vi "Servo MSMT SpecAn Create Evaluations.vi"(8 "error in (no error)":errorcluster, 11 "Servo MSMT in":refnum<class "Servo MSMT.lvclass">) -> (0 "error out":errorcluster, 2 "Specan Evaluations":T1[](array[typedef]) {"Low Limit" format="%#_13g"; "SI Scaling" items=["femto"=-15, "pico"=-12, "nano"=-9, "micro"=-6, "milli"=-3, "percent"=-2, ""=0, "kilo"=3, "mega"=6, "giga"=9, "tera"=12]}, 3 "Servo MSMT out":refnum<class "Servo MSMT.lvclass">)   [LabVIEW 2018, in "Servo MSMT.lvlib" / "Servo MSMT.lvclass"]
uses:
  Servo MSMT.lvclass
  C:/Sequence Automation/Plugins/Measurement Interface.lvlibp/Measurement Interface.lvclass
  Plugins/TestStand API Tools (TSAT).lvlibp/Evaluation Actions/Includes/Controls/TSAT Evaluation.ctl
  Plugins/TestStand API Tools (TSAT).lvlibp/Evaluation Actions/Includes/Controls/TSAT Eval SI Unit Scaling.ctl
  Plugins/TestStand API Tools (TSAT).lvlibp/Evaluation Actions/Includes/Controls/TSAT Evaluation Type.ctl
  Plugins/SeqAuto IEvaluation.lvlibp/SeqAuto IEvaluation.lvclass
  Servo MSMT.lvclass/Servo MSMT.ctl
  Protected Methods/Read DC Pins.vi
  Protected Methods/Read Servo Measurements.vi
  Plugins/SeqAuto Evaluations.lvlibp/LTE Evaluations/LTE_ACP/LTE_ACP.lvclass
  C:/Sequence Automation/Plugins/SeqAuto IEvaluation.lvlibp/SeqAuto IEvaluation.lvclass
  Plugins/SeqAuto Evaluations.lvlibp/LTE Evaluations/LTE_OBW/LTE_OBW.lvclass
  Plugins/SeqAuto Evaluations.lvlibp/SpecAn Evaluations/SpecAn CHP/SpecAn_CHP.lvclass
  Evaluations/SpecAn Evaluations/SpecAn AMPM/SpecAn_AMPM.lvclass
  Plugins/SeqAuto Evaluations.lvlibp/LTE Evaluations/LTE_SEM/LTE_SEM.lvclass
  Plugins/SeqAuto Evaluations.lvlibp/Servo/Servo Gain/Servo Gain.lvclass
  Plugins/SeqAuto Evaluations.lvlibp/PA Evaluations/PAE/PAE.lvclass
  Plugins/SeqAuto Evaluations.lvlibp/LTE Evaluations/LTE_ModAcc/LTE_ModAcc.lvclass
  Plugins/SeqAuto Evaluations.lvlibp/SpecAn Evaluations/SpecAn IM3/SpecAn_IM3.lvclass
  Plugins/SeqAuto Evaluations.lvlibp/DC Evaluations/DC_IDD.lvclass
  Plugins/Measurement Interface.lvlibp/Private Methods/Measurement Name/Read Measurement Name.vi
  Plugins/Measurement Interface.lvlibp/Private Methods/Measurement Parameters/Read Measurement Parameters.vi
  Plugins/String Database.lvlibp/String Database.lvclass
  Plugins/Test Number and Bin Generator.lvlibp/Test Number and Bin Generator/Test Number and Bin Generator.lvclass
  Plugins/TestStand API Tools (TSAT).lvlibp/Evaluation Actions/TSAT Evaluation Actions.lvlib
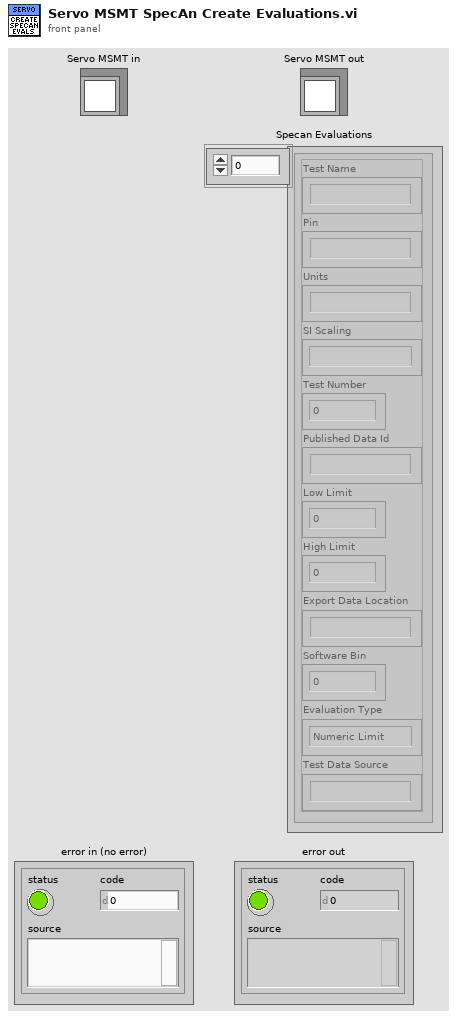
[diagram p1: front panel]
types:
  T1 = typedef "TestStand API Tools (TSAT).lvlibp/TSAT Evaluation Actions.lvlib/TSAT Evaluation.ctl" = cluster{"Test Name":string, "Pin":string, "Units":string, "SI Scaling":T2, "Test Number":i32, "Published Data Id":string, "Low Limit":dbl, "High Limit":dbl, "Export Data Location":string, "Software Bin":i64, "Evaluation Type":T3, "Test Data Source":string}
  T2 = typedef "TestStand API Tools (TSAT).lvlibp/TSAT Evaluation Actions.lvlib/TSAT Eval SI Unit Scaling.ctl" = i16
  T3 = typedef "TestStand API Tools (TSAT).lvlibp/TSAT Evaluation Actions.lvlib/TSAT Evaluation Type.ctl" = enum16{"Numeric Limit", "Pass/Fail", "None"}
  T4 = typedef "Test Number and Bin Generator.lvlibp/Test Number and Bin Generator.lvclass/Session Handle.ctl" = refnum<data-value>
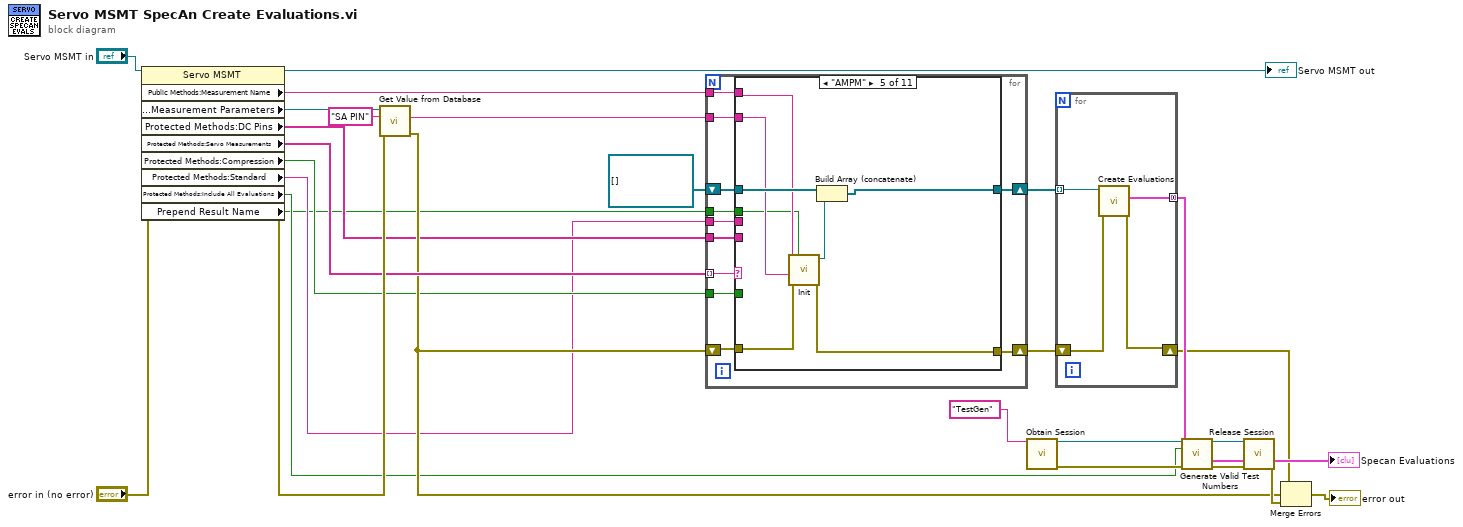
[diagram p0: block diagram]
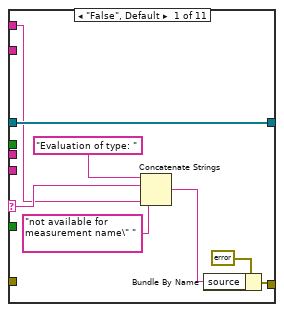
[diagram p2: hidden frame]
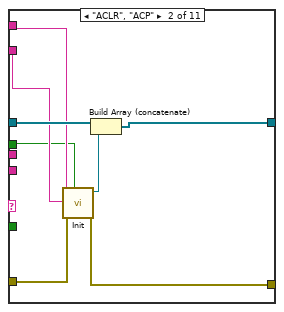
[diagram p3: hidden frame]
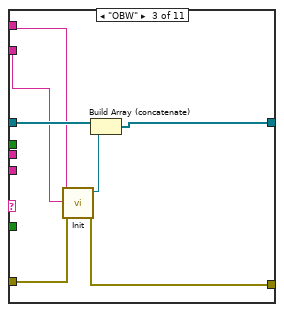
[diagram p4: hidden frame]
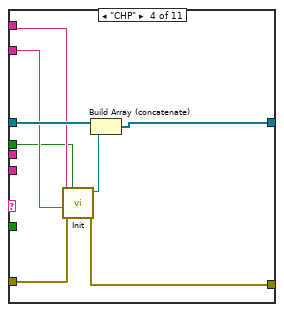
[diagram p5: hidden frame]
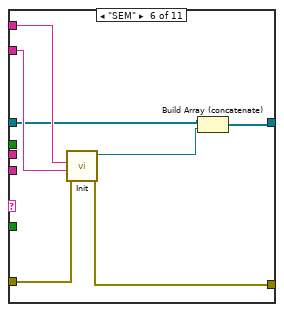
[diagram p6: hidden frame]
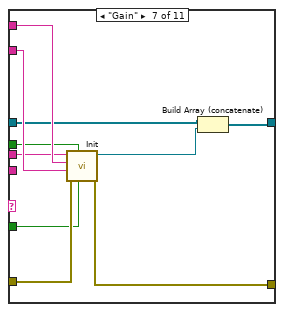
[diagram p7: hidden frame]
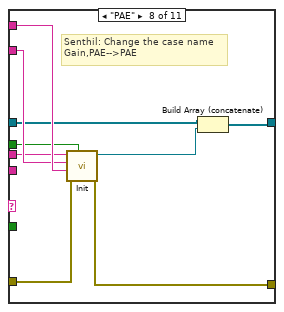
[diagram p8: hidden frame]
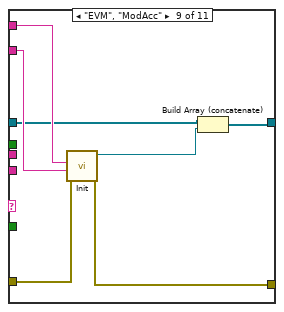
[diagram p9: hidden frame]
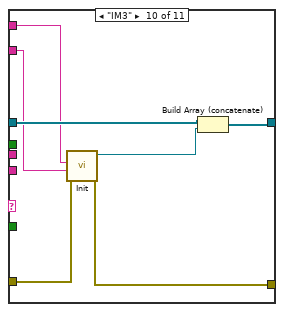
[diagram p10: hidden frame]
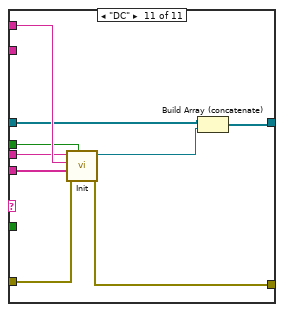
[diagram p11: hidden frame]
diagram:
  n1 = property class="Servo MSMT"(reference="Servo MSMT in", error in="error in (no error)") -> (reference out=→"Servo MSMT out":refnum<class "Servo MSMT.lvclass">, error out=w12:errorcluster, "Public Methods:Measurement Name"=w14:string, "Protected Methods:Measurement Parameters"=w18:refnum<class "String Database.lvclass">, "Protected Methods:DC Pins"=w5:string[], "Protected Methods:Servo Measurements"=w9:string[], "Protected Methods:Compression"=w4:bool, "Protected Methods:Standard"=w3:string, "Protected Methods:Include All Evaluations"=w2:bool, "Prepend Result Name"=w1:bool)
  n2 = call "Get Value from Database.vi"("error in (no error)"=w12, "Entry Name"="SA PIN", "Message in"=w18) -> ("error out"=w8:errorcluster, "Entry Value"=w17:string)  [unwired: 5 in, 2 out]
  n3 = for {
    tunnel: w17 -> [w39]
    tunnel: w14 -> [w38]
    shift-right: [w36] -> w16
    shift-left: refnum<class "SeqAuto IEvaluation.lvclass">[] [] -> [w37]
    tunnel: w9 -> [w35] mode=indexing
    shift-right: [w33] -> w7
    shift-left: w8 -> [w34]
    tunnel: w5 -> [w32]
    tunnel: w3 -> [w31]
    tunnel: w4 -> [w30]
    tunnel: w1 -> [w29]
    n4 = case shown="\"AMPM\"" w35 {
      selector: w35 -> [w43 _ _ _ _ _ _ _ _ _ _]
      tunnel: w39 -> [_ w49 w56 w64 w72 w84 w94 w103 w110 w112 _]
      tunnel: w38 -> [w41 w50 w57 w65 w73 w85 w95 w104 w111 w113 w127]
      tunnel: [w47 w55 w62 w70 w78 w79 w89 w98 w105 w114 w122] -> w36
      tunnel: w37 -> [w47 w54 w61 w69 w77 w81 w91 w100 w107 w116 w124]
      tunnel: w34 -> [_ w52 w59 w67 w75 w83 w93 w102 w109 w118 w126]
      tunnel: [w45 w51 w58 w66 w74 w82 w92 w101 w108 w117 w125] -> w33
      tunnel: w32 -> [_ _ _ _ _ _ _ _ _ _ w121]
      tunnel: w31 -> [_ _ _ _ _ _ w88 w97 _ _ w120]
      tunnel: w30 -> [_ _ _ _ _ _ w87 _ _ _ _]
      tunnel: w29 -> [_ w48 _ w63 w71 _ w86 w96 _ _ w119]
      frame "False", Default {
        n5 = Concatenate Strings("Evaluation of type: " ("source"), w43, "not available for measurement name\" " ("source"), w41) -> (w40:string)
        n6 = Bundle By Name(cluster=errorcluster {"status"=TRUE, "code"=7777, "source"=""} ("error out"), "source"=w40) -> (w45:errorcluster)
      }
      frame "ACLR", "ACP" {
        n7 = call "Init.vi"("Prepend Result Name"=w48, "error in (no error)"=w52, "SA Pin"=w49, "Measurement Name"=w50) -> ("error out"=w51:errorcluster, "LTE_ACP out"=w53:refnum<class "LTE_ACP.lvclass">)  [unwired: 6 in]
        n8 = Build Array (concatenate)(w54, w53) -> (w55:refnum<class "SeqAuto IEvaluation.lvclass">[])
      }
      frame "OBW" {
        n9 = call "Init.vi"("error in (no error)"=w59, "SA Pin"=w56, "Measurement Name"=w57) -> ("error out"=w58:errorcluster, "LTE_OBW out"=w60:refnum<class "LTE_OBW.lvclass">)  [unwired: 7 in]
        n10 = Build Array (concatenate)(w61, w60) -> (w62:refnum<class "SeqAuto IEvaluation.lvclass">[])
      }
      frame "CHP" {
        n11 = call "Init.vi"("Prepend Result Name"=w63, "error in (no error)"=w67, "SA Pin"=w64, "Measurement Name"=w65) -> ("error out"=w66:errorcluster, "SpecAn_CHP out"=w68:refnum<class "SpecAn_CHP.lvclass">)  [unwired: 6 in]
        n12 = Build Array (concatenate)(w69, w68) -> (w70:refnum<class "SeqAuto IEvaluation.lvclass">[])
      }
      frame "AMPM" {
        n13 = call "Init.vi"("Prepend Result Name"=w71, "error in (no error)"=w75, "SA Pin"=w72, "Measurement Name"=w73) -> ("error out"=w74:errorcluster, "SpecAn_AMPM out"=w76:refnum<class "SpecAn_AMPM.lvclass">)  [unwired: 6 in]
        n14 = Build Array (concatenate)(w77, w76) -> (w78:refnum<class "SeqAuto IEvaluation.lvclass">[])
      }
      frame "SEM" {
        n15 = call "Init.vi"("error in (no error)"=w83, "SA Pin"=w84, "Measurement Name"=w85) -> ("error out"=w82:errorcluster, "LTE_SEM out"=w80:refnum<class "LTE_SEM.lvclass">)  [unwired: 7 in]
        n16 = Build Array (concatenate)(w81, w80) -> (w79:refnum<class "SeqAuto IEvaluation.lvclass">[])
      }
      frame "Gain" {
        n17 = call "Init.vi"("Compression?"=w87, "Prepend Result Name"=w86, "error in (no error)"=w93, "SA Pin"=w94, "Measurement Name"=w95, "Standard"=w88) -> ("error out"=w92:errorcluster, "Servo Gain out"=w90:refnum<class "Servo Gain.lvclass">)  [unwired: 4 in]
        n18 = Build Array (concatenate)(w91, w90) -> (w89:refnum<class "SeqAuto IEvaluation.lvclass">[])
      }
      frame "PAE" {
        # "Senthil: Change the case name\nGain,PAE-->PAE"
        n19 = call "Init.vi"("Prepend Result Name"=w96, "error in (no error)"=w102, "Measurement Name"=w104, "SA Pin"=w103, "Standard"=w97) -> ("error out"=w101:errorcluster, "PAE out"=w99:refnum<class "PAE.lvclass">)  [unwired: 5 in]
        n20 = Build Array (concatenate)(w100, w99) -> (w98:refnum<class "SeqAuto IEvaluation.lvclass">[])
      }
      frame "EVM", "ModAcc" {
        n21 = call "Init.vi"("error in (no error)"=w109, "SA Pin"=w110, "Measurement Name"=w111) -> ("error out"=w108:errorcluster, "LTE_ModAcc out"=w106:refnum<class "LTE_ModAcc.lvclass">)  [unwired: 7 in]
        n22 = Build Array (concatenate)(w107, w106) -> (w105:refnum<class "SeqAuto IEvaluation.lvclass">[])
      }
      frame "IM3" {
        n23 = call "Init.vi"("error in (no error)"=w118, "SA Pin"=w112, "Measurement Name"=w113) -> ("error out"=w117:errorcluster, "SpecAn_IM3 out"=w115:refnum<class "SpecAn_IM3.lvclass">)  [unwired: 7 in]
        n24 = Build Array (concatenate)(w116, w115) -> (w114:refnum<class "SeqAuto IEvaluation.lvclass">[])
      }
      frame "DC" {
        n25 = call "Init.vi"("Prepend Result Name"=w119, "error in (no error)"=w126, "DC Pins"=w121, "Measurement Name"=w127, "Standard"=w120) -> ("error out"=w125:errorcluster, "DC_IDD out"=w123:refnum<class "DC_IDD.lvclass">)  [unwired: 5 in]
        n26 = Build Array (concatenate)(w124, w123) -> (w122:refnum<class "SeqAuto IEvaluation.lvclass">[])
      }
    }
  }
  n27 = call "Obtain Session.vi"("Session  Name ()"="TestGen") -> ("Session Handle"=w24:T4, "error out"=w21:errorcluster)  [unwired: 13 in]
  n28 = for {
    tunnel: w16 -> [w131] mode=indexing
    tunnel: [w130] -> w15 mode=concatenating
    shift-right: [w128] -> w6
    shift-left: w7 -> [w129]
    n29 = call-dynamic "Create Evaluations.vi"("error in (no error)"=w129, "IEvaluation in"=w131) -> ("error out"=w128:errorcluster, "Evaluations Out"=w130:T1[])  [unwired: 7 in, 1 out]
  }
  n30 = call "Generate Valid Test Numbers.vi"("Session Handle in"=w24, "Include All Evaluations?"=w2, "Evaluations In"=w15, "error in (no error)"=w21) -> ("Session Handle out"=w23:T4, "Evaluations Out"=→"Specan Evaluations":T1[], "error out"=w22:errorcluster)  [unwired: 9 in]
  n31 = call "Release Session.vi"("Session Handle"=w23, "error in (no error)"=w22) -> ("error out"=w11:errorcluster)  [unwired: 13 in]
  n32 = Merge Errors(w6, w8, w11) -> (→"error out":errorcluster)
